vi "Send Time Fix.vi"(6 "Current Send":u32, 9 "Last Send":u32, 11 "Spare":i32) -> (3 "Fixed Delay":i32)   [LabVIEW 2011, in "CAN FD.lvlib"]
uses:
  CAN FD.lvlib
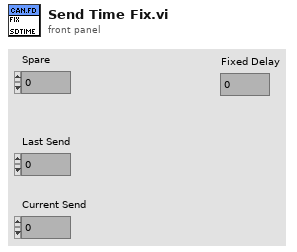
[diagram p1: front panel]
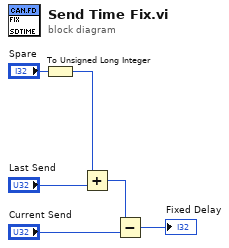
[diagram p0: block diagram]
diagram:
  n1 = To Unsigned Long Integer(number="Spare") -> (unsigned 32bit integer=w4:u32)
  n2 = Add(x=w4, y="Last Send") -> (x+y=w3:u32)
  n3 = Subtract(x=w3, y="Current Send") -> (x-y=→"Fixed Delay":u32)
